vi "Launch Config Manager.vi"(8 "error in (no error)":errorcluster, 11 "VolatusCore in":refnum<class "VolatusCore.lvclass">) -> (0 "error out":errorcluster, 3 "VolatusCore out":refnum<class "VolatusCore.lvclass">)   [LabVIEW 2020, in "Volatus.lvlib" / "VolatusCore.lvclass"]
uses:
  VolatusCore.lvclass
  VolatusCore.lvclass/VolatusCore.ctl
  ConfigAPI/ConfigAPI.lvclass/ConfigAPI.ctl
  lv-promises/Promises/Promise/Promise.lvclass/Promise.ctl
  lv-promises/Promises/Future/Future.lvclass/Future.ctl
  VolatusConfigManager Messages/Load Config Msg/Load Config Msg.lvclass/Load Config Msg.ctl
  <vilib>/ActorFramework/Message Enqueuer/Message Enqueuer.lvclass/Message Enqueuer.ctl
  App/App.lvclass/App.ctl
  Event Level.ctl
  VolatusConfigManager Messages/Load Config Msg/Send Load Config.vi
  lv-promises/Promises/Promise/Future.vi
  <vilib>/ActorFramework/Message Enqueuer/Enqueue.vi
  VolatusConfigTask/VolatusConfigManager.lvclass
  C:/dev/lv20CE/relink/lv-volatus/Volatus/Task/Task.lvclass
  VolatusNodeValue/VolatusNodeValue.lvclass
  C:/dev/lv20CE/relink/lv-promises/Promises/Value/Value.lvclass
  VolatusConfigManager Messages/Load Config Msg/Load Config Msg.lvclass
  C:/Program Files (x86)/National Instruments/LabVIEW 2020/vi.lib/ActorFramework/Message/Message.lvclass
  <vilib>/ActorFramework/Message Priority Queue/Priority Enqueue.vi
  lv-promises/Promises/Future/Wait.vi
  VolatusNodeValue/Read.vi
  lv-promises/Promises/Future/Future.lvclass
  App/App.lvclass
  Volatus.lvlib
  ConfigAPI/ConfigAPI.lvclass
  VolatusConfig/Node/Node.lvclass
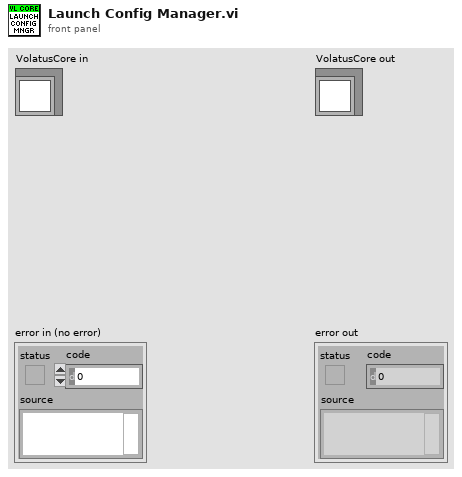
[diagram p1: front panel]
types:
  T1 = typedef "Volatus.lvlib/Event Level.ctl" = enum16{"Debug", "Info", "Warning", "Error"}
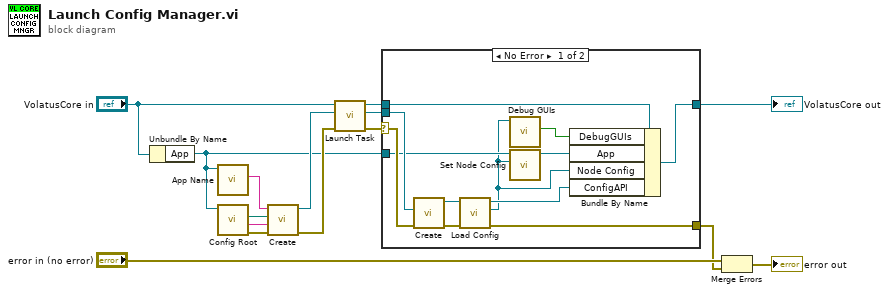
[diagram p0: block diagram]
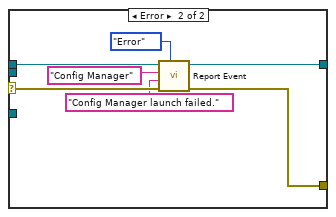
[diagram p2: hidden frame]
diagram:
  n1 = Unbundle By Name("VolatusCore in") -> ("App"=w1:refnum<class "App.lvclass">)
  n2 = call-dynamic "App Name.vi"("App in"=w1) -> ("App Name"=w2:string)  [unwired: 10 in]
  n3 = call-dynamic "Config Root.vi"("App in"=w1) -> ("error out"=w6:errorcluster, "Main Filename"=w5:string, "Config Root"=w7:path)  [unwired: 7 in, 1 out]
  n4 = call "Create.vi"("error in (no error)"=w6, "Main Filename"=w5, "Config Root"=w7, "Node Name"=w2) -> ("error out"=w3:errorcluster, "VolatusConfig out"=w4:refnum<class "VolatusConfigManager.lvclass">)  [unwired: 6 in]
  n5 = call "Launch Task.vi"("error in (no error)"=w3, "Task"=w4, "VolatusCore in"="VolatusCore in") -> ("error out"=w14:errorcluster, "EnQr"=w9:refnum<class "Message Enqueuer.lvclass">, "VolatusCore out"=w15:refnum<class "VolatusCore.lvclass">)  [unwired: 6 in]
  n6 = case shown="No Error" w14 {
    selector: w14 -> [w26 w33]
    tunnel: w15 -> [w25 w34]
    tunnel: [w21 w30] -> w11
    tunnel: [w24 w29] -> w10
    tunnel: w9 -> [w27 _]
    tunnel: w1 -> [w20 _]
    frame No Error {
      n7 = call "Create.vi"("error in (no error)"=w26, "EnQr"=w27) -> ("error out"=w22:errorcluster, "ConfigAPI out"=w23:refnum<class "ConfigAPI.lvclass">)  [unwired: 8 in]
      n8 = call "Load Config.vi"("error in (no error)"=w22, "ConfigAPI in"=w23) -> ("error out"=w21:errorcluster, "Node"=w17:refnum<class "Node.lvclass">, "ConfigAPI out"=w18:refnum<class "ConfigAPI.lvclass">)  [unwired: 7 in]
      n9 = call "Debug GUIs.vi"("Node in"=w17) -> ("DebugGUIs"=w16:bool)  [unwired: 8 in, 2 out]
      n10 = call "Set Node Config.vi"("Node Config"=w17, "App in"=w20) -> ("App out"=w19:refnum<class "App.lvclass">)  [unwired: 8 in, 1 out]
      n11 = Bundle By Name(cluster=w25, "DebugGUIs"=w16, "App"=w19, "Node Config"=w17, "ConfigAPI"=w18) -> (w24:refnum<class "VolatusCore.lvclass">)
    }
    frame Error {
      n12 = call "Report Event.vi"("Level (Info)"=Event_Level."Error", "error in (no error)"=w33, "Message"="Config Manager launch failed.", "Context"="Config Manager", "VolatusCore in"=w34) -> ("error out"=w30:errorcluster, "VolatusCore out"=w29:refnum<class "VolatusCore.lvclass">)  [unwired: 5 in]
    }
  }
  "VolatusCore out" <- w10
  n13 = Merge Errors("error in (no error)", w11) -> (→"error out":errorcluster)
